vi "Chamber controller June 30 2016 TEMP.vi"() -> ()   [LabVIEW 2014]
uses:
  <vilib>/Instr/_visa.llb/VISA Configure Serial Port (Instr).vi
  Environmental Chamber LabVIEW and Instruments/Drivers and Software/Keithley 2100 Series/Public/Configure/Configure 2 Wire Resistance.vi
  <vilib>/Utility/file.llb/Write To Spreadsheet File (string).vi
  <vilib>/Utility/file.llb/Read From Spreadsheet File (string).vi
  Environmental Chamber LabVIEW and Instruments/Drivers and Software/keithley_6430/Keithley 6430/Public/Data/Read (Single Point).vi
  Environmental Chamber LabVIEW and Instruments/Drivers and Software/LabVIEW 8.2 Drivers/keithley_24xx/Keithley 24XX/Public/Data/Read (Single Point).vi
  Environmental Chamber LabVIEW and Instruments/Drivers and Software/keithley_24xx/Keithley 24XX/Keithley 24XX.lvlib
  Environmental Chamber LabVIEW and Instruments/Drivers and Software/keithley_6430/Keithley 6430/Keithley 6430.lvlib
  Environmental Chamber LabVIEW and Instruments/Drivers and Software/Keithley 2100 Series/Keithley 2100 Series.lvlib
panel:
  out "Current setpoint (C)":dbl
  in  "J-KEM temp control cluster":T1 {"Set temp (C)" min=0.0 max=130.0}
  out "saving data?":bool
  out "ArduinoQCM\ncluster":T2 caption="Arduino QCM" {"Freq 5" format="%#_10g"; "Freq 4" format="%#_10g"; "Freq 3" format="%#_10g"; "Freq 2" format="%#_10g"; "Freq 1" format="%#_10g"}
  in  "Data logging settings":T3={"Save during sequence only"=TRUE, "Save now"=FALSE, "sec between data points"=0.0, "Current data file path"=path "", "Save sample names"={"QCM1"="aQCM2", "QCM2"="aQCM2", "QCM3"="aQCM3", "QCM4"="aQCM4", "QCM5"="aQCM5", "QCM6"="aQCM6", "SRS"="sample_SRS", "K-2420"="Keithley2420", "K-6430"="Keithley6430", "K-2100"="Keithley2100"}, "Experiment Notes"=""} {"sec between data points" min=0.0 max=30.0 format="%#_13g"}
  in  "Sequence cluster":T4={"Save sequence"=FALSE, "Clear sequence"=FALSE, "Import sequence file"=FALSE, "Tare elapsed time"=TRUE, "Run Sequence"=FALSE, "Stop program when sequence ends"=TRUE, "User-defined\nsequence"=[], "Sequence end time"="", "Sequence\npreview"=[]} caption="Sequence settings"
  in  "Pressure parameters cluster":T5={"valve % open"=100.0, "Desired pressure"=0.0, "Vapor sccm"=0.0, "Gas sccm"=0.0, "Valve mode"=enum."% Open", "Pressure Mode"=enum."Abs. pressure", "analyte partial pressure"=23.8, "Turbo pump\nauto on"=TRUE, "Valve position (%)"=0.0, "read pressure"=0.0, "read vapor flow"=0.0, "read gas flow"=0.0, "pressure chart"={"pressure"=0.0}} caption="Pressure settings" {"read gas flow" format="%#_3g"; "read vapor flow" format="%#_3g"; "read pressure" format="%#_7f"; "Valve position (%)" format="%#_3g"; "analyte partial pressure" min=0.0 max=100.0 step=5.0; "Gas sccm" min=0 max=200 step=5; "Vapor sccm" min=0 max=200 step=5; "Desired pressure" min=0.0 max=760.0 step=5.0; "valve % open" min=0.0 max=100.0 step=5.0 format="%#_2f"}
  out "Elapsed time (min)":dbl
  out "State date/time":string caption="Start time"
  out "K-2100 (Ohm)":cluster{"Measurement":dbl}(graph) caption="K-2100 Ohm"
  out "K-6430":cluster{"Measurement":dbl}(graph)
  out "K-2420":cluster{"Resistance":sgl}(graph)
  in  "Gate time (sec)":enum16{"0.1", "1.0 ", "10"}(ring)=enum."1.0 "
  out "MHz":dbl format="%.9f"
  out "QCM plot":T6(graph)
  in  "Stop":bool
  in  "Clear all charts":bool
  out "O2 sensor output":dbl[](array[numeric]) caption="atm\nTorr"
  in  "rapidox O2 Sensor":bool
  in  "setnag O2 Pump":bool
  in  "Baud Rate 2":i32(ring)=2 items=["2400", "4800", "9600", "19200", "38400", "57600", "115200"]
  in  "Com Port":i32(ring) items=["Com 1", "Com 2", "Com 3", "Com 4", "Com 5", "Com 6", "COM 7", "COM 8", "COM 9", "COM 10", "COM 11", "COM 12", "com 13", "COM 14"]
  in  "Com Port 2":i32(ring) items=["Com 1", "Com 2", "Com 3", "Com 4", "Com 5", "Com 6", "COM 7", "COM 8", "COM 9", "COM 10", "COM 11", "COM 12", "com 13", "COM 14"]
  out "Waveform Chart":cluster{dbl}(graph)
  out "O2 Concentration (PPM)":dbl
  out "Waveform Chart 6":cluster{dbl}(graph)
  # "Currently Unused"
  # "100%"
  # "SRS"
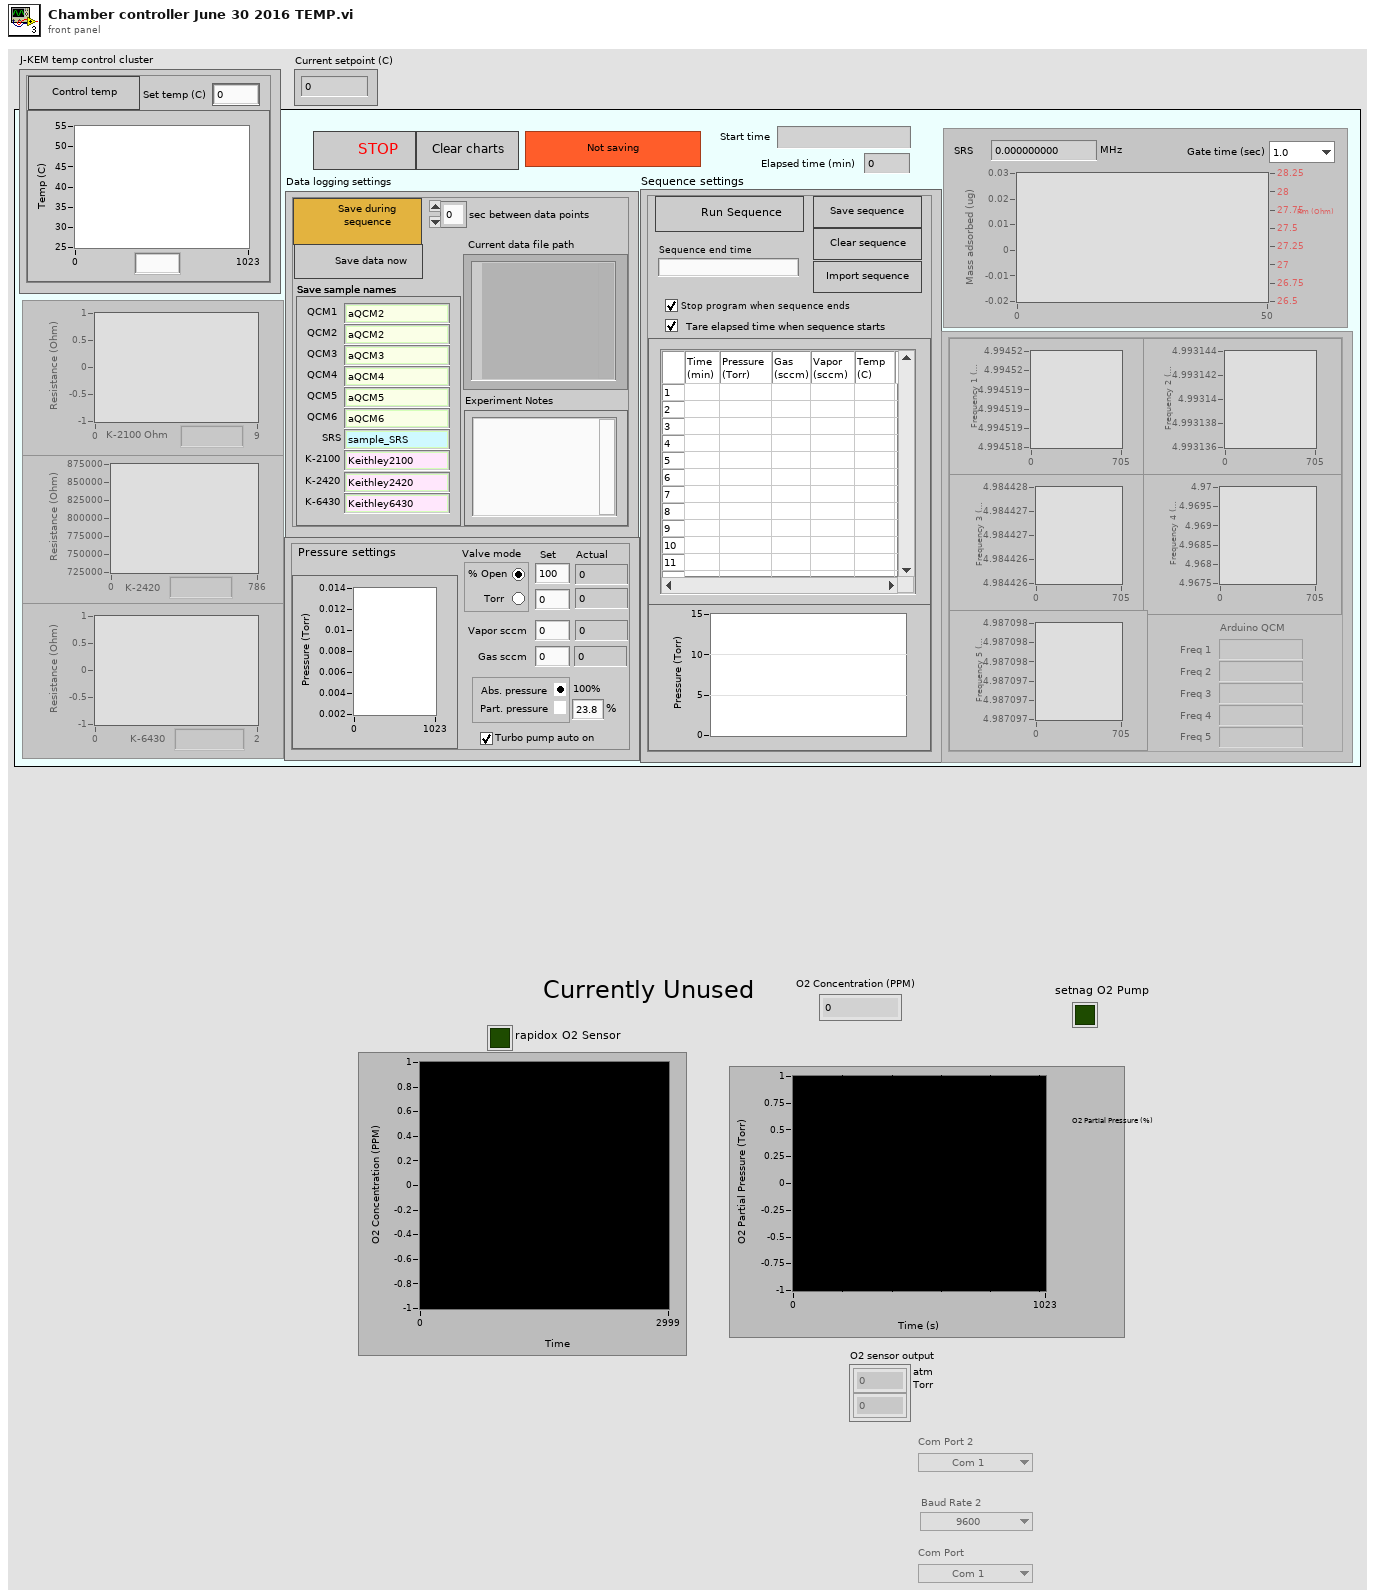
[diagram p1: front panel]
types:
  T1 = cluster{"Set temp (C)":dbl, "Control temp":bool, "J-KEM temp chart":dbl}
  T2 = cluster{"arduino qcm 1":dbl, "Freq 1":dbl, "arduino qcm 2":dbl, "Freq 2":dbl, "arduino qcm 3":dbl, "Freq 3":dbl, "arduino qcm 4":dbl, "Freq 4":dbl, "arduino qcm 5":dbl, "Freq 5":dbl}
  T3 = cluster{"Save during sequence only":bool, "Save now":bool, "sec between data points":dbl, "Current data file path":path, "Save sample names":cluster{"QCM1":string, "QCM2":string, "QCM3":string, "QCM4":string, "QCM5":string, "QCM6":string, "SRS":string, "K-2420":string, "K-6430":string, "K-2100":string}, "Experiment Notes":string}
  T4 = cluster{"Save sequence":bool, "Clear sequence":bool, "Import sequence file":bool, "Tare elapsed time":bool, "Run Sequence":bool, "Stop program when sequence ends":bool, "User-defined\nsequence":string[][], "Sequence end time":string, "Sequence\npreview":cluster{dbl[], dbl[]}[]}
  T5 = cluster{"valve % open":dbl, "Desired pressure":dbl, "Vapor sccm":sgl, "Gas sccm":sgl, "Valve mode":enum32{"% Open", "Torr "}, "Pressure Mode":enum32{"Abs. pressure", " Part. pressure"}, "analyte partial pressure":dbl, "Turbo pump\nauto on":bool, "Valve position (%)":dbl, "read pressure":dbl, "read vapor flow":dbl, "read gas flow":dbl, "pressure chart":cluster{"pressure":dbl}}
  T6 = cluster{"Numeric Control":dbl, "Resistance out":dbl}
  T7 = cluster{"Keithley 6430":bool, "J-KEM":bool, "Keithley 2420":bool, "Keithley 2100":bool, "SRS QCM":bool, "Pressure control":bool, "Arduino":bool}
  T8 = enum8{"Enabled", "Disabled", "Disabled and Grayed Out"}
  T9 = cluster{"Arduino 1":refnum<visa-resource-name>, "Arduino 2":refnum<visa-resource-name>, "Arduino 3":refnum<visa-resource-name>, "Arduino 4":refnum<visa-resource-name>, "Arduino 5":refnum<visa-resource-name>}
  T10 = enum16{"open", "open or create", "create or replace", "create", "open (read only)"}
  T11 = enum16{"no parity", "odd parity", "even parity", "mark parity", "space parity"}
  T12 = cluster{"f":dbl, "f":dbl, "f":dbl, "f":dbl, "f":dbl}
  T13 = cluster{"String":string, "String":string, "String":string}
  T14 = cluster{"task out":refnum<k21>, "error out":errorcluster, "task out":refnum<k21>, "error out":errorcluster, "task out":refnum<k21>, "error out":errorcluster, "VISA resource name":refnum<visa-resource-name>, "error out":errorcluster}
  T15 = cluster{"task out":refnum<k21>, "error out":errorcluster, "task out":refnum<k21>, "error out":errorcluster, "task out":refnum<k21>, "error out":errorcluster, "VISA resource name out":refnum<visa-resource-name>, "error out":errorcluster}
  T16 = cluster{bool, "VISA resource name":refnum<visa-resource-name>, "error out":errorcluster}
  T17 = cluster{bool, "VISA resource name out":refnum<visa-resource-name>, "error out":errorcluster}
  T18 = cluster{"VISA resource name out":refnum<visa-resource-name>, "error out":errorcluster, "VISA resource name out":refnum<visa-resource-name>, "error out":errorcluster, "VISA resource name out":refnum<visa-resource-name>, "error out":errorcluster, "VISA resource name out":refnum<visa-resource-name>, "error out":errorcluster, "VISA resource name out":refnum<visa-resource-name>, "error out":errorcluster}
  T19 = cluster{bool, cluster{"task out":refnum<k21>, "error out":errorcluster, "task out":refnum<k21>, "error out":errorcluster, "task out":refnum<k21>, "error out":errorcluster, "VISA resource name out":refnum<visa-resource-name>, "error out":errorcluster}}
  T20 = cluster{bool, "VISA out":refnum<visa-resource-name>, "error out":errorcluster}
  T21 = cluster{"Boolean":bool, "VISA out":refnum<visa-resource-name>, "error out":errorcluster}
  T22 = cluster{"Numeric Control":dbl, "Cluster":cluster{"Numeric Control":dbl}, "String":string, "error out":errorcluster}
  T23 = cluster{bool, "Com Port":i32, "Numeric Control out":dbl}
  T24 = cluster{"VISA Refnum out":refnum<visa-resource-name>, "error out":errorcluster, "VISA Refnum out":refnum<visa-resource-name>, "error out":errorcluster, "VISA Refnum out":refnum<visa-resource-name>, "error out":errorcluster, "VISA Refnum out":refnum<visa-resource-name>, "error out":errorcluster, "VISA Refnum out":refnum<visa-resource-name>, "error out":errorcluster}
  T25 = cluster{"f":string, "f":string, "f":string, "f":string, "f":string}
  T26 = cluster{"valve % open":dbl, "Desired pressure":dbl, "Vapor sccm":sgl, "Gas sccm":sgl, "Valve mode":enum32{"% Open", "Torr "}, "Pressure Mode":enum32{"Abs. pressure", " Part. pressure"}, "analyte partial pressure":dbl, "Turbo pump\nauto on":bool}
  T27 = cluster{"User-defined\nsequence":string[][], "Present (s)":dbl, "current  step # in":i32, "sequence end time in":timestamp}
  T28 = cluster{"current  step # in":i32, "sequence end time in":timestamp, "Boolean":bool}
  T29 = cluster{"press/RH/gas/vapor":cluster{"pressure":string, "RH":string, "gas flow":string, "vapor flow":string}, "Cluster":cluster{"Valve position (%)":dbl, "read pressure":dbl, "read vapor flow":dbl, "read gas flow":dbl}}
  T30 = cluster{"Boolean":bool, "DAQ IDs in":cluster{"task out":refnum<k21>, "error out":errorcluster, "task out":refnum<k21>, "error out":errorcluster, "task out":refnum<k21>, "error out":errorcluster, "VISA Refnum out":refnum<visa-resource-name>, "error out":errorcluster}}
  T31 = cluster{"Boolean":bool, "VISA resource name out":refnum<visa-resource-name>, "error out":errorcluster}
  T32 = cluster{"current temp string":string, string, string, string}
  T33 = cluster{"f":dbl, "f":dbl, "f":dbl, "f":dbl, "f":dbl}[]
  T34 = cluster{"pressure":string, "RH":string, "gas flow":string, "vapor flow":string}
  T35 = cluster{"Valve position (%)":dbl, "read pressure":dbl, "read vapor flow":dbl, "read gas flow":dbl}
  T36 = cluster{"f":dbl, "f":dbl, "f":dbl, "f":dbl, "f":dbl, "f":dbl, "f":dbl, "f":dbl, "f":dbl, "f":dbl}
  T37 = cluster{"QCM1":string, "QCM2":string, "QCM3":string, "QCM4":string, "QCM5":string, "QCM6":string, "SRS":string, "K-2420":string, "K-6430":string, "K-2100":string}
  T38 = cluster{"task out":refnum<k21>, "error out":errorcluster, "task out":refnum<k21>, "error out":errorcluster, "task out":refnum<k21>, "error out":errorcluster, "VISA Refnum out":refnum<visa-resource-name>, "error out":errorcluster}
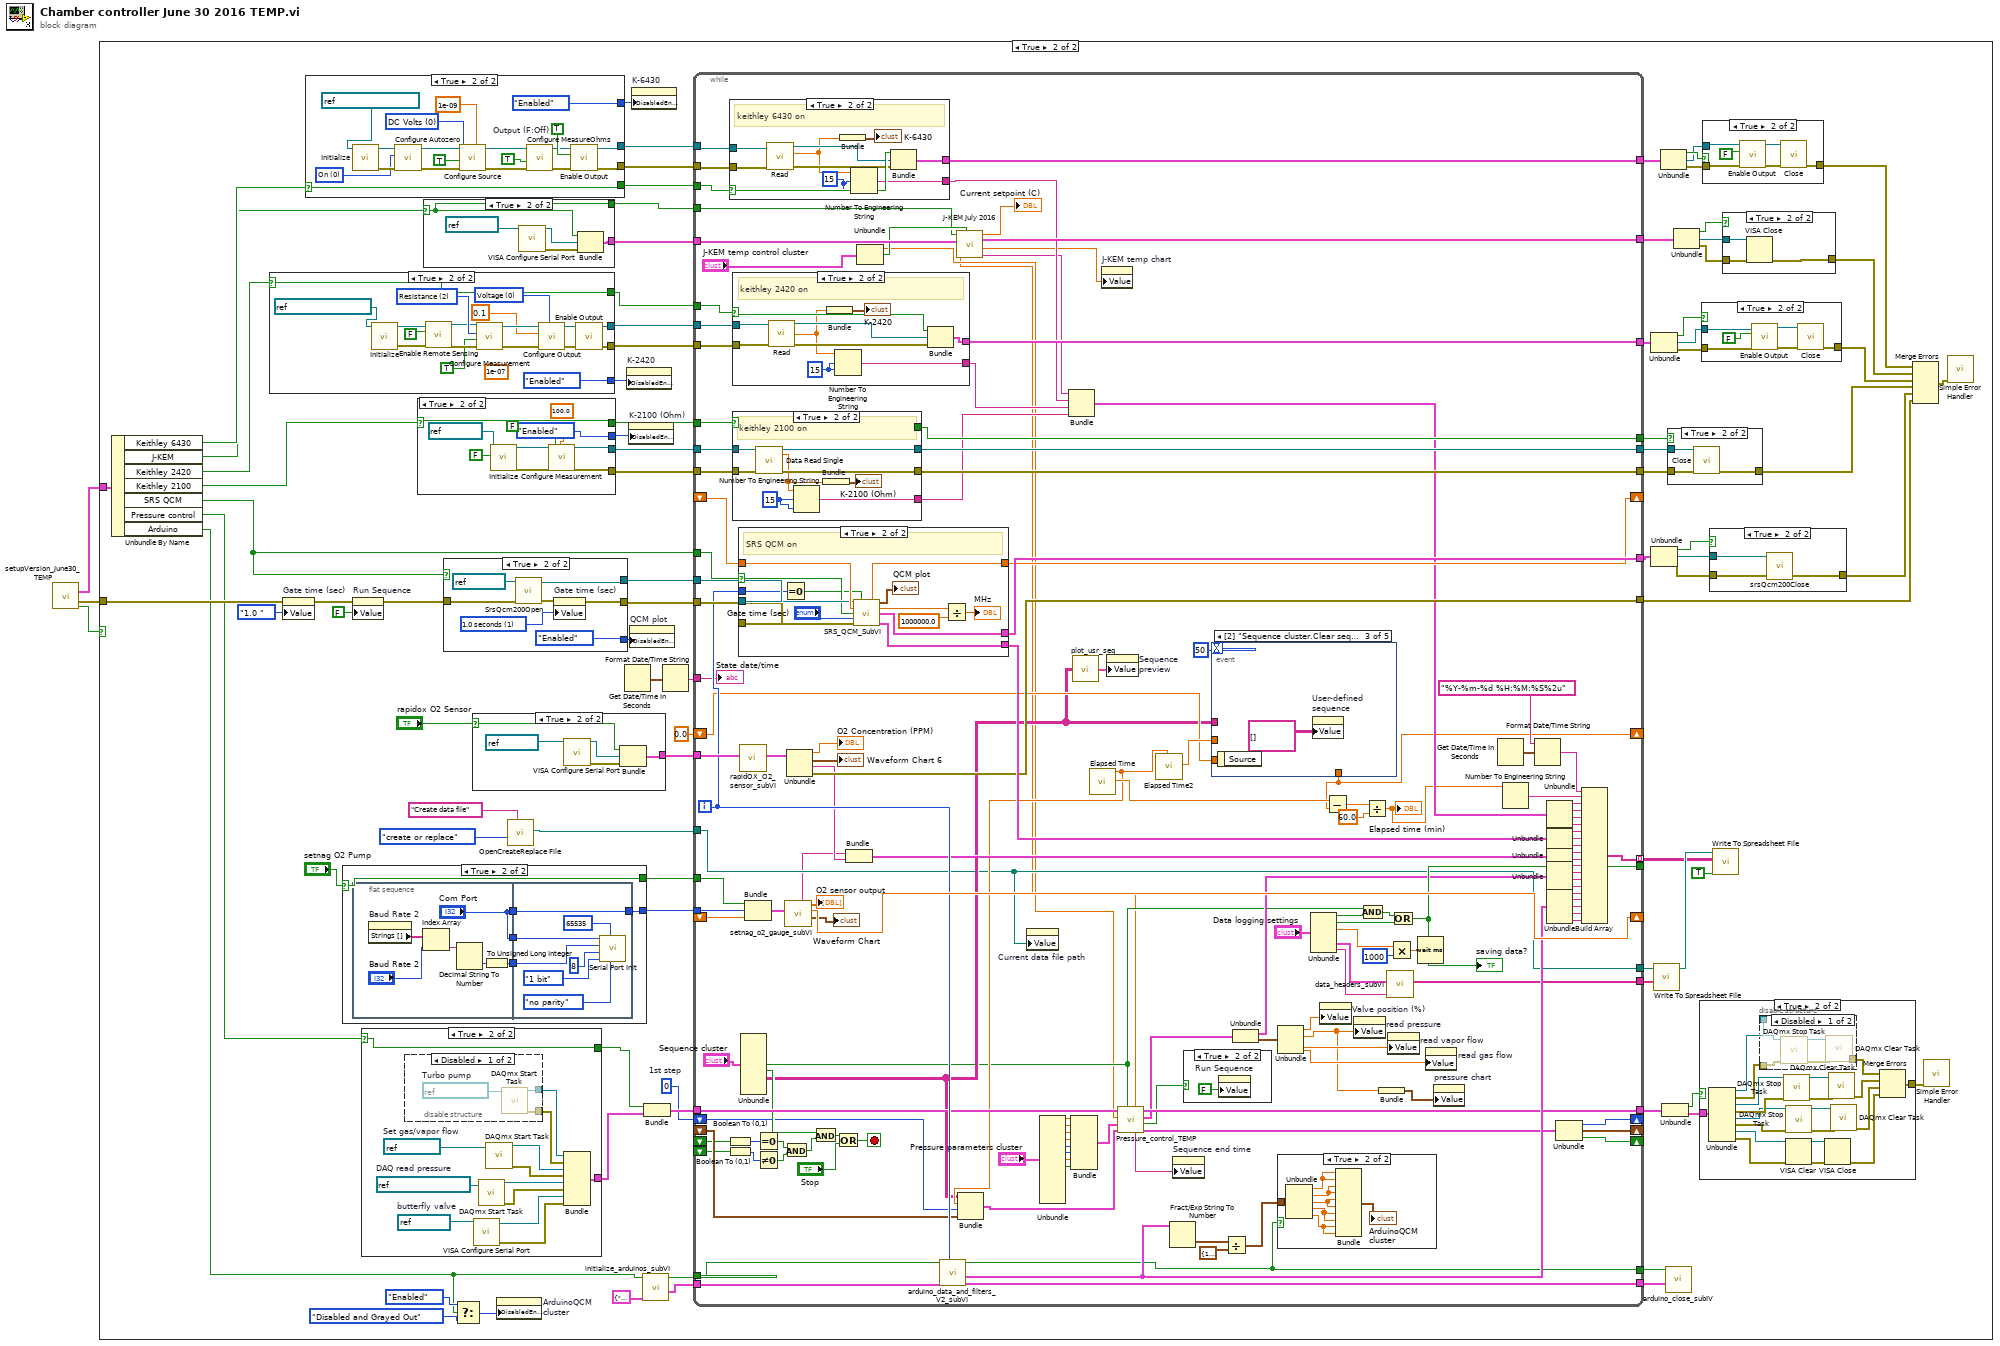
[diagram p0: block diagram]
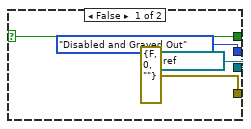
[diagram p4: hidden frame]
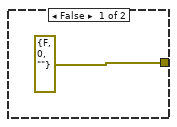
[diagram p5: hidden frame]
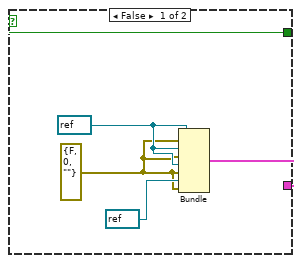
[diagram p7: hidden frame]
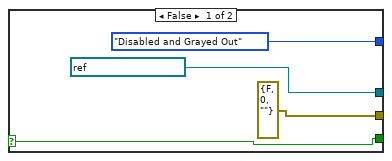
[diagram p10: hidden frame]
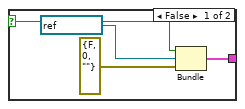
[diagram p11: hidden frame]
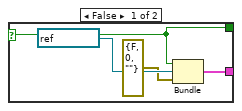
[diagram p13: hidden frame]
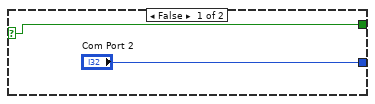
[diagram p14: hidden frame]
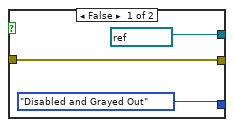
[diagram p16: hidden frame]
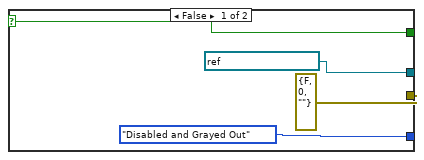
[diagram p18: hidden frame]
diagram:
  n1 = call "setupVersion_June30_TEMP.vi"() -> ("Instruments on/off"=w1:T7, "error IO"=w2:errorcluster, "OK"=w3:bool)  [unwired: 13 in]
  n2 = case shown="True" w3 {
    tunnel: w2 -> [_ w12]
    tunnel: w1 -> [_ w11]
    frame False {
    }
    frame True {
      w24 = 0  # 1st step
      n3 = Unbundle By Name(w11) -> ("Keithley 6430"=w10:bool, "J-KEM"=w9:bool, "Keithley 2420"=w8:bool, "Keithley 2100"=w7:bool, "SRS QCM"=w6:bool, "Pressure control"=w5:bool, "Arduino"=w4:bool)
      n4 = case shown="True" w8 {
        selector: w8 -> [w250 w254]
        tunnel: [refnum<visa-resource-name> "GPIB1::24::INSTR" ("VISA resource name") w263] -> w89
        tunnel: [errorcluster {"status"=FALSE, "code"=0, "source"=""} ("error out") w258] -> w88
        tunnel: [T8."Disabled and Grayed Out" ("Disabled") T8."Enabled" ("Disabled")] -> w52
        tunnel: [w250 w254] -> w45
        frame False {
        }
        frame True {
          (unwired) 1e-07 ("Manual Range (1.0)")
          w265 = u16 0 items=["Voltage", "Current"] ("Source Mode  (0: Voltage)")
          w270 = u16 2 items=["Volts", "Current", "Resistance"] ("Function (0: Volts)")
          n5 = call "Initialize.vi"("VISA resource name"=refnum<visa-resource-name> "GPIB1::24::INSTR") -> ("error out"=w259:errorcluster, "VISA resource name out"=w262:refnum<visa-resource-name>)  [unwired: 9 in]
          n6 = call "Enable Remote Sensing.vi"("error in (no error)"=w259, "Enable Remote Sensing (T: Enable)"=FALSE ("4-wire?"), "VISA resource name"=w262) -> ("error out"=w260:errorcluster, "VISA resource name out"=w261:refnum<visa-resource-name>)  [unwired: 7 in]
          n7 = call "Configure Measurement.vi"("error in (no error)"=w260, "Enable Auto Range (T:Enable)"=TRUE, "Function (0: Volts)"=w270, "VISA resource name"=w261) -> ("error out"=w269:errorcluster, "VISA resource name out"=w268:refnum<visa-resource-name>)  [unwired: 6 in]
          n8 = call "Configure Output.vi"("Source Mode  (0: Voltage)"=w265, "error in (no error)"=w269, "Output Level (0)"=0.1 ("Applied Voltage (V)"), "VISA resource name"=w268) -> ("error out"=w267:errorcluster, "VISA resource name out"=w266:refnum<visa-resource-name>)  [unwired: 6 in]
          n9 = call "Enable Output.vi"("error in (no error)"=w267, "VISA resource name"=w266) -> ("error out"=w258:errorcluster, "VISA resource name out"=w263:refnum<visa-resource-name>)  [unwired: 8 in]
        }
      }
      n10 = property on="Gate time (sec)" class="Enum (strict)"(error in=w12, "Value"=enum16{"0.1", "1.0 ", "10"}."1.0 " ("Gate time (sec)")) -> (error out=w13:errorcluster)  [unwired: 1 in, 1 out]
      n11 = case shown="True" w10 {
        selector: w10 -> [w164 w168]
        tunnel: [refnum<visa-resource-name> "GPIB0::29::INSTR" ("VISA resource name") w181] -> w58
        tunnel: [errorcluster {"status"=FALSE, "code"=0, "source"=""} ("error out") w182] -> w57
        tunnel: [T8."Disabled and Grayed Out" ("Disabled") T8."Enabled" ("Disabled")] -> w51
        tunnel: [w164 w168] -> w44
        frame False {
        }
        frame True {
          w170 = u16 0 items=["DC Volts", "DC Current"] ("Source Function (0: DC Volts)")
          w177 = u16 0 items=["On", "Off", "Once"] ("Autozero  (0: On)")
          w185 = TRUE  # Output (F:Off)
          n12 = call "Initialize.vi"("VISA resource name"=refnum<visa-resource-name> "GPIB0::30::INSTR") -> ("error out"=w178:errorcluster, "VISA resource name out"=w179:refnum<visa-resource-name>)  [unwired: 4 in, 5 out]
          n13 = call "Configure Autozero.vi"("error in (no error)"=w178, "Autozero  (0: On)"=w177, "VISA resource name"=w179) -> ("error out"=w173:errorcluster, "VISA resource name out"=w175:refnum<visa-resource-name>)  [unwired: 7 in]
          n14 = call "Configure Source.vi"("I-Source Level [A]"=1e-09, "error in (no error)"=w173, "Auto Range (T:Enable)"=TRUE, "Source Function (0: DC Volts)"=w170, "VISA resource name"=w175) -> ("error out"=w172:errorcluster, "VISA resource name out"=w174:refnum<visa-resource-name>)  [unwired: 5 in]
          n15 = call "Configure MeasureOhms.vi"("error in (no error)"=w172, "Auto Range (T:Enable)"=TRUE, "VISA resource name"=w174) -> ("error out"=w186:errorcluster, "VISA resource name out"=w184:refnum<visa-resource-name>)  [unwired: 3 in, 4 out]
          n16 = call "Enable Output.vi"("error in (no error)"=w186, "Enable Output (F:Off)"=w185, "VISA resource name"=w184) -> ("error out"=w182:errorcluster, "VISA resource name out"=w181:refnum<visa-resource-name>)  [unwired: 7 out]
        }
      }
      n17 = case shown="True" "setnag O2 Pump" {
        selector: "setnag O2 Pump" -> [w209 w211]
        tunnel: ["Com Port 2" w212] -> w85
        tunnel: [w209 w211] -> w33
        frame False {
        }
        frame True {
          n18 = flat-sequence {
            tunnel: ["Com Port"] -> w215
            tunnel: [w217] -> w214
            tunnel: ["Com Port"] -> w213
            tunnel: w215 -> [w223]
            tunnel: w214 -> [w222]
            tunnel: w213 -> [w224]
            tunnel: [w224] -> w212
            frame #0 {
              n19 = property on="Baud Rate 2" class="Ring (strict)"() -> ("Strings []"=w219:string[])  [unwired: 2 in, 2 out]
              n20 = Index Array(array=w219, index="Baud Rate 2") -> (element=w220:string)
              n21 = Decimal String To Number(string=w220) -> (number=w218:i32)  [unwired: 2 in, 1 out]
              n22 = To Unsigned Long Integer(number=w218) -> (unsigned 32bit integer=w217:u32)
            }
            frame #1 {
              n23 = call <vilib>:"Serial Port Init.vi"("parity"=T11."no parity", "buffer size"=u16 65535, "stop bits"=enum16{"1 bit", "1.5 bits", "2 bits"}."1 bit", "data bits"=u16 8, "baud rate"=w222, "port number"=w223) -> ()  [unwired: 1 in, 1 out]
            }
          }
        }
      }
      n24 = property on="Run Sequence" class="Bool (strict)"(error in=w13, "Value"=FALSE) -> (error out=w19:errorcluster)  [unwired: 1 in, 1 out]
      n25 = case shown="True" w5 {
        selector: w5 -> [w136 w141]
        tunnel: [w137 w143] -> w26
        tunnel: [w136 w141] -> w27
        frame False {
          w139 = refnum<k21> refnum ("task out")
          w138 = errorcluster {"status"=FALSE, "code"=0, "source"=""} ("error out")
          n26 = Bundle("task out"=w139, "error out"=w138, "task out"=w139, "error out"=w138, "task out"=w139, "error out"=w138, "VISA resource name"=refnum<visa-resource-name> refnum, "error out"=w138) -> (w137:T14)  [unwired: 1 in]
        }
        frame True {
          w151 = refnum<visa-resource-name> "COM5"  # butterfly valve
          w152 = refnum<k21> "Setflow"  # Set gas/vapor flow
          w153 = refnum<k21> "AllDaqReadings"  # DAQ read pressure
          n27 = disable-structure shown="Disabled" {
            disable-tunnel: [w155 _] -> w150
            disable-tunnel: [w154 _] -> w149
            frame Disabled {
              w156 = refnum<k21> "TurboON"  # Turbo pump
              n28 = call <vilib>:"DAQmx Start Task.vi"("task/channels in"=w156) -> ("task out"=w155:refnum<k21>, "error out"=w154:errorcluster)  [unwired: 13 in]
            }
            frame Enabled {
            }
          }
          n29 = call-poly "VISA Configure Serial Port"("VISA resource name"=w151) -> ("VISA resource name out"=w144:refnum<visa-resource-name>, "error out"=w142:errorcluster)  [unwired: 13 in]
          n30 = call <vilib>:"DAQmx Start Task.vi"("task/channels in"=w153) -> ("task out"=w146:refnum<k21>, "error out"=w145:errorcluster)  [unwired: 13 in]
          n31 = call <vilib>:"DAQmx Start Task.vi"("task/channels in"=w152) -> ("task out"=w148:refnum<k21>, "error out"=w147:errorcluster)  [unwired: 13 in]
          n32 = Bundle("task out"=w150, "error out"=w149, "task out"=w148, "error out"=w147, "task out"=w146, "error out"=w145, "VISA resource name out"=w144, "error out"=w142) -> (w143:T15)  [unwired: 1 in]
        }
      }
      n33 = case shown="True" w7 {
        selector: w7 -> [w97 w103]
        tunnel: [refnum<visa-resource-name> "K-2100" ("VISA resource name out") w106] -> w42
        tunnel: [errorcluster {"status"=FALSE, "code"=0, "source"=""} ("error out") w105] -> w41
        tunnel: [w97 w103] -> w40
        tunnel: [T8."Disabled and Grayed Out" ("Disabled") T8."Enabled" ("Disabled")] -> w35
        frame False {
        }
        frame True {
          n34 = call "Initialize.vi"("VISA resource name"=refnum<visa-resource-name> "K-2100", "Reset? (T: Reset)"=FALSE) -> ("VISA resource name out"=w107:refnum<visa-resource-name>, "error out"=w104:errorcluster)  [unwired: 16 in]
          n35 = call-poly "Configure Measurement.vi"("VISA resource name"=w107, "error in (no error)"=w104, "Auto Range? (T: Auto)"=FALSE, "Custom Range (100 Ohm)"=100.0 ("Temp (C) 2")) -> ("VISA resource name out"=w106:refnum<visa-resource-name>, "error out"=w105:errorcluster)  [unwired: 14 in]
        }
      }
      n36 = case shown="True" w9 {
        selector: w9 -> [w200 w205]
        tunnel: [w201 w206] -> w74
        tunnel: [w200 w205] -> w68
        frame False {
          n37 = Bundle(w200, "VISA resource name"=refnum<visa-resource-name> "COM3", "error out"=errorcluster {"status"=FALSE, "code"=0, "source"=""}) -> (w201:T16)  [unwired: 1 in]
        }
        frame True {
          n38 = call-poly "VISA Configure Serial Port"("VISA resource name"=refnum<visa-resource-name> "COM3") -> ("VISA resource name out"=w207:refnum<visa-resource-name>, "error out"=w204:errorcluster)  [unwired: 13 in]
          n39 = Bundle(w205, "VISA resource name out"=w207, "error out"=w204) -> (w206:T17)  [unwired: 1 in]
        }
      }
      n40 = case shown="True" w6 {
        tunnel: [refnum<visa-resource-name> "COM6" ("VISA in") w239] -> w87
        tunnel: [w234 w236] -> w86
        tunnel: w19 -> [w234 w241]
        tunnel: [T8."Disabled and Grayed Out" ("Disabled") T8."Enabled" ("Disabled")] -> w53
        frame False {
        }
        frame True {
          w238 = u16 1 items=["0.1 seconds", "1.0 seconds", "10.0 seconds"] ("Gate time")
          n41 = call "SrsQcm200Open.vi"("error in"=w241, "VISA in"=refnum<visa-resource-name> "COM6") -> ("error out"=w237:errorcluster, "VISA out"=w239:refnum<visa-resource-name>)  [unwired: 3 in]
          n42 = property on="Gate time (sec)" class="Enum (strict)"(error in=w237, "Value"=w238) -> (error out=w236:errorcluster)  [unwired: 1 in, 1 out]
        }
      }
      n43 = Select(t=T8."Enabled" ("Disabled"), s=w4, f=T8."Disabled and Grayed Out" ("Disabled")) -> (s? t:f=w18:T8)
      n44 = case shown="True" "rapidox O2 Sensor" {
        selector: "rapidox O2 Sensor" -> [w187 w192]
        tunnel: [w188 w193] -> w64
        frame False {
          n45 = Bundle(w187, "VISA resource name"=refnum<visa-resource-name> "COM7", "error out"=errorcluster {"status"=FALSE, "code"=0, "source"=""}) -> (w188:T16)  [unwired: 1 in]
        }
        frame True {
          n46 = call-poly "VISA Configure Serial Port"("VISA resource name"=refnum<visa-resource-name> "COM7") -> ("VISA resource name out"=w194:refnum<visa-resource-name>, "error out"=w191:errorcluster)  [unwired: 13 in]
          n47 = Bundle(w192, "VISA resource name out"=w194, "error out"=w191) -> (w193:T17)  [unwired: 1 in]
        }
      }
      n48 = property on="ArduinoQCM\ncluster" class="Clust (strict)"("DisabledEnum"=w18) -> ()  [unwired: 2 in, 2 out]
      n49 = call "OpenCreateReplace File.vi"("prompt"="Create data file", "function (open:0)"=T10."create or replace") -> ("new file path"=w43:path)  [unwired: 6 in, 3 out]
      n50 = Get Date/Time In Seconds() -> (seconds since 1Jan1904=w91:timestamp)
      n51 = property on="K-2420" class="WFChart (strict)"("DisabledEnum"=w52) -> ()  [unwired: 2 in, 2 out]
      n52 = property on="K-2100 (Ohm)" class="WFChart (strict)"("DisabledEnum"=w35) -> ()  [unwired: 2 in, 2 out]
      n53 = property on="QCM plot" class="WFChart (strict)"("DisabledEnum"=w53) -> ()  [unwired: 2 in, 2 out]
      n54 = property on="K-6430" class="WFChart (strict)"("DisabledEnum"=w51) -> ()  [unwired: 2 in, 2 out]
      n55 = call "initialize_arduinos_subVI.vi"("arduino 1-6 addresses"=T9 {"Arduino 1"="COM21", "Arduino 2"="COM22", "Arduino 3"="COM23", "Arduino 4"="COM24", "Arduino 5"="COM26"}, "arduinos on?"=w4) -> ("arduino addresses/errors"=w28:T18, "arduinos on/off"=w49:bool)  [unwired: 8 in]
      n56 = Bundle(w27, w26) -> (w25:T19)  [unwired: 1 in]
      n57 = Format Date/Time String(seconds (now)=w91) -> (date/time string=w32:string)  [unwired: 2 in]
      n58 = while {
        shift-right: [w418] -> _
        shift-left: _ -> [w340]
        tunnel: [w403] -> w50 mode=indexing if=w366
        tunnel: w45 -> [w408]
        tunnel: w89 -> [w417]
        tunnel: w88 -> [w416]
        tunnel: w87 -> [w415]
        tunnel: w86 -> [w414]
        tunnel: w6 -> [w413]
        tunnel: w33 -> [w342]
        tunnel: w85 -> [w343]
        tunnel: [w412] -> w82
        tunnel: [w411] -> w78
        tunnel: w74 -> [w410]
        tunnel: [w409] -> w73
        tunnel: w68 -> [w275]
        tunnel: w64 -> [w354]
        tunnel: [w350] -> w30
        tunnel: [w282] -> w63
        tunnel: w43 -> [w282]
        shift-right: [w401] -> _
        shift-left: _ -> [w402]
        tunnel: w58 -> [w407]
        tunnel: w57 -> [w406]
        tunnel: [w405] -> w56
        tunnel: [w366] -> _
        tunnel: w49 -> [w349]
        tunnel: w28 -> [w394]
        tunnel: [w348] -> w47
        tunnel: [w393] -> w48
        tunnel: [w385] -> w46
        tunnel: w44 -> [w378]
        tunnel: w42 -> [w365]
        tunnel: w41 -> [w364]
        tunnel: w40 -> [w363]
        tunnel: [w362] -> w39
        tunnel: [w361] -> w38
        tunnel: [w360] -> w37
        shift-right: [w334] -> _
        shift-left: 0.0 ("Elapsed Time (s)") -> [w335]
        tunnel: w32 -> [w325]
        tunnel: w25 -> [w307]
        shift-right: [w302] -> _
        shift-left: w24 -> [w295]
        shift-right: [w301] -> _
        shift-left: _ -> [w299]
        shift-right: [w300] -> _
        shift-left: _ -> [w298]
        shift-left: _ -> [w297]
        tunnel: [w293] -> w23
        i -> [w344]
        stop <- w368 stop-if-true
        n59 = Boolean To (0,1)(Boolean=w298) -> (0, 1=w376:i16)
        n60 = Boolean To (0,1)(Boolean=w297) -> (0, 1=w375:i16)
        n61 = case "Keithley 6430" shown="True" w378 {
          selector: w378 -> [w452 w463]
          tunnel: w407 -> [w451 w460]
          tunnel: w406 -> [w450 w459]
          tunnel: ["" w462] -> w347
          tunnel: [w449 w461] -> w405
          frame False {
            # "keithley 6430 off"
            n62 = Bundle(w452, "VISA resource name out"=w451, "error out"=w450) -> (w449:T17)  [unwired: 1 in]
          }
          frame True {
            w454 = i16 15 ("width (-)")
            # "keithley 6430 on"
            n63 = call-poly "Read.vi"("error in (no error)"=w459, "VISA resource name"=w460) -> ("error out"=w458:errorcluster, "Measurement"=w456:dbl, "VISA resource name out"=w457:refnum<visa-resource-name>)  [unwired: 1 in, 6 out]
            n64 = Bundle("Measurement"=w456) -> (→"K-6430":cluster{"Measurement":dbl})  [unwired: 1 in]
            n65 = Number To Engineering String(2:w454, 3:w454, 4:w456) -> (0:w462:string)  [unwired: 1 in]
            n66 = Bundle(w463, "VISA resource name out"=w457, "error out"=w458) -> (w461:T17)  [unwired: 1 in]
          }
        }
        n67 = case shown="True" w363 {
          selector: w363 -> [w428 w433]
          tunnel: [w429 w440] -> w361
          tunnel: [w430 w439] -> w360
          tunnel: w365 -> [w429 w438]
          tunnel: w364 -> [w430 w437]
          tunnel: ["" w435] -> w345
          tunnel: [w428 w433] -> w362
          frame False {
            # "keithley 2100 off"
          }
          frame True {
            w432 = i16 15 ("width (-)")
            # "keithley 2100 on"
            n68 = call "Data Read Single.vi"("VISA resource name"=w438, "error in (no error)"=w437) -> ("VISA resource name out"=w440:refnum<visa-resource-name>, "Measurement"=w436:dbl, "error out"=w439:errorcluster)  [unwired: 15 in]
            n69 = Number To Engineering String ("elapsed time (min)")(2:w432, 3:w432, 4:w436) -> (0:w435:string)  [unwired: 1 in]
            n70 = Bundle("Measurement"=w436) -> (→"K-2100 (Ohm)":cluster{"Measurement":dbl})  [unwired: 1 in]
          }
        }
        n71 = case "Keithley 2420" shown="True" w408 {
          selector: w408 -> [w467 w476]
          tunnel: w417 -> [w466 w471]
          tunnel: w416 -> [w465 w470]
          tunnel: [w464 w474] -> w412
          tunnel: ["" w473] -> w346
          frame False {
            # "keithley 2420 off"
            n72 = Bundle(w467, "VISA resource name out"=w466, "error out"=w465) -> (w464:T17)  [unwired: 1 in]
          }
          frame True {
            w469 = i16 15 ("width (-)")
            # "keithley 2420 on"
            n73 = call-poly "Read.vi"("VISA resource name"=w471, "error in (no error)"=w470) -> ("VISA resource name out"=w477:refnum<visa-resource-name>, "Resistance"=w472:sgl, "error out"=w475:errorcluster)  [unwired: 7 in, 4 out]
            n74 = Bundle("Resistance"=w472) -> (→"K-2420":cluster{"Resistance":sgl})  [unwired: 1 in]
            n75 = Number To Engineering String(2:w469, 3:w469, 4:w472) -> (0:w473:string)  [unwired: 1 in]
            n76 = Bundle(w476, "VISA resource name out"=w477, "error out"=w475) -> (w474:T17)  [unwired: 1 in]
          }
        }
        n77 = case "SRS QCM" shown="True" w413 {
          selector: w413 -> [w481 w492]
          tunnel: w415 -> [w484 w494]
          tunnel: w414 -> [w483 w495]
          tunnel: [w482 w498] -> w411
          tunnel: w402 -> [w479 w497]
          tunnel: [w479 w496] -> w401
          tunnel: [T13 {"String"="", "String"="", "String"=""} ("M,F,MR output cluster") w491] -> w391
          tunnel: w344 -> [_ w485]
          frame False {
            # "SRS QCM off"
            n78 = Bundle(w481, "VISA out"=w484, "error out"=w483) -> (w482:T20)  [unwired: 1 in]
          }
          frame True {
            # "SRS QCM on"
            n79 = Equal To 0?(x=w485) -> (x = 0?=w486:bool)
            n80 = call "SRS_QCM_SubVI.vi"("VISA Refnum in"=w494, "first iteration?"=w486, "Frequency out 3"=w497, "Boolean 2"=w492, "Gate time"="Gate time (sec)", "error in (no error)"=w495) -> ("Frequency out 2"=w496:dbl, "Cluster"=→"QCM plot":T6, "Frequency out"=w487:dbl, "Cluster 2"=w498:T21, "M,F,MR output cluster"=w491:T13)  [unwired: 2 in, 3 out]
            n81 = Divide(x=w487, y=1000000.0) -> (x/y=→"MHz":dbl)
          }
        }
        n82 = call "rapidOX_O2_sensor_subVI.vi"("rapid ox info in"=w354) -> ("rapidox info out"=w353:T22)  [unwired: 10 in]
        n83 = Unbundle("Sequence cluster") -> ("Run Sequence"=w287:bool, "Stop program when sequence ends"=w296:bool, "User-defined\nsequence"=w291:string[][])  [unwired: 6 out]
        n84 = Bundle(w342, "Com Port"=w343, "Numeric Control out"=w340) -> (w341:T23)  [unwired: 1 in]
        n85 = Equal To 0?(x=w376) -> (x = 0?=w373:bool)
        n86 = Not Equal To 0?(x=w375) -> (x != 0?=w374:bool)
        n87 = And(x=w373, y=w374) -> (x .and. y?=w367:bool)
        n88 = call "setnag_o2_gauge_subVI.vi"("setnag info in"=w341) -> ("Cluster"=→"Waveform Chart":cluster{"Numeric Control":dbl}, "Numeric Control out"=w418:dbl, "Array"=→"O2 sensor output":dbl[], "String"=w279:string)  [unwired: 7 in]
        n89 = Unbundle(w353) -> ("Numeric Control"=→"O2 Concentration (PPM)":dbl, "Cluster"=→"Waveform Chart 6":cluster{"Numeric Control":dbl}, "String"=w324:string, "error out"=w350:errorcluster)
        n90 = And(x=w296, y=w367) -> (x .and. y?=w338:bool)
        n91 = Or(x=w338, y="Stop") -> (x .or. y?=w368:bool)
        n92 = Bundle("String"=w279, "String"=w324) -> (w323:cluster{"String":string, "String":string})  [unwired: 1 in]
        n93 = Unbundle("J-KEM temp control cluster") -> ("Set temp (C)"=w273:dbl, "Control temp"=w276:bool)  [unwired: 1 out]
        n94 = call "arduino_data_and_filters_V2_subVI.vi"("loop iteration number"=w344, "arduino 1-6 address and errors"=w394, "arduinos on?"=w349) -> ("arduino 1-6 addresses and errors out"=w393:T24, "arduino 1-6 data out"=w392:T25, "arduinos on? output"=w348:bool)  [unwired: 6 in]
        n95 = property on="Current data file path" class="Path"("Value"=w282) -> ()  [unwired: 2 in, 2 out]
        n96 = Unbundle("Pressure parameters cluster") -> ("valve % open"=w312:dbl, "Desired pressure"=w314:dbl, "Vapor sccm"=w315:sgl, "Gas sccm"=w316:sgl, "Valve mode"=w317:enum32{"% Open", "Torr "}, "Pressure Mode"=w318:enum32{"Abs. pressure", " Part. pressure"}, "analyte partial pressure"=w319:dbl, "Turbo pump\nauto on"=w320:bool)  [unwired: 5 out]
        n97 = Bundle("valve % open"=w312, "Desired pressure"=w314, "Vapor sccm"=w315, "Gas sccm"=w316, "Valve mode"=w317, "Pressure Mode"=w318, "analyte partial pressure"=w319, "Turbo pump\nauto on"=w320) -> (w311:T26)  [unwired: 1 in]
        n98 = call "plot_usr_seq.vi"("User-defined sequence"=w291) -> ("Sequence Preview"=w283:cluster{dbl[], dbl[]}[])
        n99 = call "Elapsed Time"() -> ("Present (s)"=w304:dbl, "Elapsed Time (s)"=w356:dbl)  [unwired: 12 in, 6 out]
        n100 = Bundle("User-defined\nsequence"=w291, "Present (s)"=w304, "current  step # in"=w295, "sequence end time in"=w299) -> (w305:T27)  [unwired: 1 in]
        n101 = property on="Sequence\npreview" class="XYGraph (strict)"("Value"=w283) -> ()  [unwired: 2 in, 2 out]
        n102 = call "Pressure_control_TEMP.vi"("Run Sequence"=w287, "user sequence, present (s) in, current step in, seq time in"=w305, "pressure parameters in"=w311, "set temp"=w273, "pressure control on? / DAQ IDs/errors in"=w307) -> ("current step # out, shift register time out, seq button on?"=w303:T28, "sequence over? USE THIS TO REINITIALIZE RUN SEQUENCE BUTTON SO PROGRAM ENDS"=w292:bool, "save press/RH/gasflow/vaporflow - read valve position/pressure/vaporflow/gasflow"=w290:T29, "pressure control on out, DAQ IDs/errors out"=w293:T30, "sequence end date/time string"=w294:string, "Temp setpoint"=w272:dbl)  [unwired: 1 in]
        n103 = call "J-KEM July 2016.vi"("Control temp?"=w276, "Set temp (C)"=w272, "Address in"=w410, "J-KEM on?"=w275) -> ("current temp string"=w333:string, "Current temp (C)"=w277:dbl, "Address out"=w409:T31, "Current setpoint (C)"=→"Current setpoint (C)":dbl)  [unwired: 4 in]
        n104 = Bundle("current temp string"=w333, w347, w346, w345) -> (w339:T32)  [unwired: 1 in]
        n105 = property on="J-KEM temp chart" class="WFChart (strict)"("Value"=w277) -> ()  [unwired: 2 in, 2 out]
        n106 = call "Elapsed Time2"("Set Start Time (s)"=w304) -> ("Elapsed Time (s)"=w336:dbl)  [unwired: 11 in, 7 out]
        n107 = Fract/Exp String To Number(string=w392) -> (number=w384:T12)  [unwired: 3 in, 1 out]
        n108 = property on="Sequence end time" class="Str"("Value"=w294) -> ()  [unwired: 2 in, 2 out]
        n109 = case shown="True" w292 {
          frame False {
          }
          frame True {
            n110 = property on="Run Sequence" class="Bool (strict)"("Value"=FALSE ("Run Sequence")) -> ()  [unwired: 2 in, 2 out]
          }
        }
        n111 = event shown="[2] \"Sequence cluster.Clear sequence\": Value Change" {
          selector: _ -> [_ _ _ _ _]
          dyn-events: _ -> [_ _ _ _ _]
          timeout: 50 -> [_ _ _ _ _]
          tunnel: w291 -> [_ _ _ w447 _]
          tunnel: w336 -> [_ _ _ _ _]
          tunnel: w335 -> [w441 _ _ _ _]
          tunnel: [w441 _ _ _ _] -> w334
          event Timeout {
            n112 = event-data() -> ()  [unwired: 1 in, 1 out]
          }
          event "Clear all charts": Value Change {
            (unwired) T33 [] ("History Data")
            w444 = cluster{dbl}[] [] ("History Data")
            w445 = cluster{"Resistance":sgl}[] [] ("History Data")
            w443 = dbl[] [] ("History Data")
            n113 = event-data() -> ()  [unwired: 1 in, 1 out]
            n114 = property on="K-6430" class="WFChart (strict)"("History Data"=w445) -> ()  [unwired: 2 in, 2 out]
            n115 = property on="arduino qcm 3" class="WFChart (strict)"("History Data"=w443) -> ()  [unwired: 2 in, 2 out]
            n116 = property on="arduino qcm 1" class="WFChart (strict)"("History Data"=w443) -> ()  [unwired: 2 in, 2 out]
            n117 = property on="Waveform Chart" class="WFChart (strict)"("History Data"=w444) -> ()  [unwired: 2 in, 2 out]
            n118 = property on="QCM plot" class="WFChart (strict)"("History Data"=cluster{dbl, "Resistance out":dbl}[] []) -> ()  [unwired: 2 in, 2 out]
            n119 = property on="K-2100 (Ohm)" class="WFChart (strict)"("History Data"=w445) -> ()  [unwired: 2 in, 2 out]
            n120 = property on="arduino qcm 4" class="WFChart (strict)"("History Data"=w443) -> ()  [unwired: 2 in, 2 out]
            n121 = property on="K-2420" class="WFChart (strict)"("History Data"=w445) -> ()  [unwired: 2 in, 2 out]
            n122 = property on="pressure chart" class="WFChart (strict)"("History Data"=w444) -> ()  [unwired: 2 in, 2 out]
            n123 = property on="arduino qcm 2" class="WFChart (strict)"("History Data"=w443) -> ()  [unwired: 2 in, 2 out]
            n124 = property on="arduino qcm 5" class="WFChart (strict)"("History Data"=w443) -> ()  [unwired: 2 in, 2 out]
          }
          event "Sequence cluster.Clear sequence": Value Change {
            n125 = event-data() -> ()  [unwired: 1 in, 1 out]
            n126 = property on="User-defined\nsequence" class="Tbl (strict)"("Value"=string[][] []) -> ()  [unwired: 2 in, 2 out]
          }
          event "Sequence cluster.Save sequence": Value Change {
            n127 = event-data() -> ()  [unwired: 1 in, 1 out]
            n128 = call-poly <vilib>:"Write To Spreadsheet File.vi"("2D data"=w447) -> ()  [unwired: 7 in, 1 out]
          }
          event "Sequence cluster.Import sequence file": Value Change {
            n129 = event-data() -> ()  [unwired: 1 in, 1 out]
            n130 = call-poly <vilib>:"Read From Spreadsheet File.vi"() -> ("all rows"=w448:string[][])  [unwired: 7 in, 4 out]
            n131 = property on="User-defined\nsequence" class="Tbl (strict)"("Value"=w448) -> ()  [unwired: 2 in, 2 out]
          }
        }
        n132 = Divide(x=w384, y=T12 {"f"=1000000.0, "f"=1000000.0, "f"=1000000.0, "f"=1000000.0, "f"=1000000.0}) -> (x/y=w359:T12)
        n133 = Unbundle(w290) -> ("press/RH/gas/vapor"=w289:T34, "Cluster"=w288:T35)
        n134 = Unbundle(w288) -> ("Valve position (%)"=w286:dbl, "read pressure"=w281:dbl, "read vapor flow"=w285:dbl, "read gas flow"=w284:dbl)
        n135 = case shown="True" w348 {
          tunnel: w359 -> [_ w427]
          frame False {
          }
          frame True {
            n136 = Unbundle(w427) -> ("f"=w426:dbl, "f"=w425:dbl, "f"=w424:dbl, "f"=w423:dbl, "f"=w422:dbl)
            n137 = Bundle("f"=w426, "f"=w426, "f"=w425, "f"=w425, "f"=w424, "f"=w424, "f"=w423, "f"=w423, "f"=w422, "f"=w422) -> (→"ArduinoQCM\ncluster":T36)  [unwired: 1 in]
          }
        }
        n138 = Unbundle("Data logging settings") -> ("Save during sequence only"=w370:bool, "Save now"=w372:bool, "sec between data points"=w358:dbl, "Save sample names"=w309:T37, "Experiment Notes"=w308:string)  [unwired: 1 out]
        n139 = property on="Valve position (%)" class="DigNum (strict)"("Value"=w286) -> ()  [unwired: 2 in, 2 out]
        n140 = Subtract(x=w356, y=w334) -> (x-y=w355:dbl)
        n141 = property on="read pressure" class="DigNum (strict)"("Value"=w281) -> ()  [unwired: 2 in, 2 out]
        n142 = And(x=w287, y=w370) -> (x .and. y?=w369:bool)
        n143 = Divide(x=w355, y=60.0) -> (x/y=w326:dbl)
        "Elapsed time (min)" <- w326
        n144 = Bundle("read pressure"=w281) -> (w280:cluster{"read pressure":dbl})  [unwired: 1 in]
        n145 = call "data_headers_subVI.vi"("Experiment Notes"=w308, "Sample names"=w309) -> ("data headers"=w385:string[])  [unwired: 9 in]
        n146 = property on="read vapor flow" class="DigNum (strict)"("Value"=w285) -> ()  [unwired: 2 in, 2 out]
        n147 = Multiply(x=w358, y=u32 1000 ("x")) -> (x*y=w398:dbl)
        n148 = Or(x=w369, y=w372) -> (x .or. y?=w366:bool)
        "saving data?" <- w366
        n149 = Wait (ms)(milliseconds to wait=w398) -> ()  [unwired: 1 out]
        n150 = property on="read gas flow" class="DigNum (strict)"("Value"=w284) -> ()  [unwired: 2 in, 2 out]
        n151 = property on="pressure chart" class="WFChart (strict)"("Value"=w280) -> ()  [unwired: 2 in, 2 out]
        n152 = Get Date/Time In Seconds() -> (seconds since 1Jan1904=w419:timestamp)
        n153 = Number To Engineering String ("elapsed time (min)")(4:w326) -> (0:w331:string)  [unwired: 3 in]
        n154 = Format Date/Time String(time format string (%c)="%Y-%m-%d %H:%M:%S%2u", seconds (now)=w419) -> (date/time string=w395:string)  [unwired: 1 in]
        n155 = Unbundle(w339) -> ("current temp string"=w330:string, w329:string, w328:string, w327:string)
        n156 = Unbundle(w391) -> ("String"=w332:string, "String"=w397:string, "String"=w396:string)
        n157 = Unbundle(w323) -> ("String"=w322:string, "String"=w321:string)
        n158 = Unbundle(w289) -> ("pressure"=w382:string, "RH"=w381:string, "gas flow"=w380:string, "vapor flow"=w379:string)
        n159 = Unbundle ("arduino 1-6")(w392) -> ("f"=w390:string, "f"=w389:string, "f"=w388:string, "f"=w387:string, "f"=w386:string)
        n160 = Unbundle(w303) -> ("current  step # in"=w302:i32, "sequence end time in"=w301:timestamp, "Boolean"=w300:bool)
        n161 = Build Array(w395, w331, w330, w329, w328, w327, w332, w397, w396, w322, w321, w382, w381, w380, w379, w390, w389, w388, w387, w386) -> (w403:string[])
        "State date/time" <- w325
      }
      n162 = Unbundle(w82) -> (w81:bool, "VISA resource name out"=w80:refnum<visa-resource-name>, "error out"=w79:errorcluster)
      n163 = Unbundle(w78) -> ("Boolean"=w77:bool, "VISA out"=w76:refnum<visa-resource-name>, "error out"=w75:errorcluster)
      n164 = call-poly <vilib>:"Write To Spreadsheet File.vi"("1D data"=w46, "file path (dialog if empty)"=w63) -> ("new file path (Not A Path if cancelled)"=w67:path)  [unwired: 6 in]
      n165 = Unbundle(w56) -> (w61:bool, "VISA resource name out"=w60:refnum<visa-resource-name>, "error out"=w59:errorcluster)
      n166 = Unbundle(w23) -> ("Boolean"=w22:bool, "DAQ IDs in"=w21:T38)
      n167 = call "arduino_close_subIV.vi"("arduino 1-6 addresses and errors out"=w48, "arduinos on?"=w47) -> ()  [unwired: 10 in]
      n168 = case shown="True" w39 {
        tunnel: w38 -> [_ w95]
        tunnel: w37 -> [w92 w94]
        tunnel: [w92 w93] -> w36
        frame False {
        }
        frame True {
          n169 = call "Close.vi"("VISA resource name"=w95, "error in (no error)"=w94) -> ("error out"=w93:errorcluster)  [unwired: 17 in]
        }
      }
      n170 = Unbundle(w73) -> ("Boolean"=w72:bool, "VISA resource name out"=w71:refnum<visa-resource-name>, "error out"=w70:errorcluster)
      n171 = case shown="True" w22 {
        tunnel: w21 -> [_ w124]
        tunnel: [errorcluster {"status"=FALSE, "code"=0, "source"=""} ("error out") w111] -> w31
        frame False {
        }
        frame True {
          n172 = Unbundle(w124) -> ("task out"=w123:refnum<k21>, "error out"=w122:errorcluster, "task out"=w121:refnum<k21>, "error out"=w120:errorcluster, "task out"=w119:refnum<k21>, "error out"=w118:errorcluster, "VISA Refnum out"=w117:refnum<visa-resource-name>, "error out"=w116:errorcluster)
          n173 = disable-structure shown="Disabled" {
            disable-tunnel: [w133 _] -> w115
            disable-tunnel: w123 -> [w132 _]
            disable-tunnel: w122 -> [w131 _]
            frame Disabled {
              n174 = call <vilib>:"DAQmx Stop Task.vi"("task/channels in"=w132, "error in"=w131) -> ("task out"=w134:refnum<k21>, "error out"=w135:errorcluster)  [unwired: 12 in]
              n175 = call <vilib>:"DAQmx Clear Task.vi"("task in"=w134, "error in"=w135) -> ("error out"=w133:errorcluster)  [unwired: 13 in]
            }
            frame Enabled {
            }
          }
          n176 = call <vilib>:"DAQmx Stop Task.vi"("task/channels in"=w121, "error in"=w120) -> ("task out"=w128:refnum<k21>, "error out"=w127:errorcluster)  [unwired: 12 in]
          n177 = call <vilib>:"DAQmx Stop Task.vi"("task/channels in"=w119, "error in"=w118) -> ("task out"=w129:refnum<k21>, "error out"=w130:errorcluster)  [unwired: 12 in]
          n178 = VISA Clear(VISA resource name=w117, error in (no error)=w116) -> (VISA resource name out=w126:refnum<visa-resource-name>, error out=w125:errorcluster)
          n179 = VISA Close(VISA resource name=w126, error in (no error)=w125) -> (error out=w112:errorcluster)
          n180 = call <vilib>:"DAQmx Clear Task.vi"("task in"=w128, "error in"=w127) -> ("error out"=w114:errorcluster)  [unwired: 13 in]
          n181 = call <vilib>:"DAQmx Clear Task.vi"("task in"=w129, "error in"=w130) -> ("error out"=w113:errorcluster)  [unwired: 13 in]
          n182 = Merge Errors(w115, w114, w113, w112) -> (w111:errorcluster)
        }
      }
      n183 = case shown="True" w81 {
        tunnel: w80 -> [_ w246]
        tunnel: w79 -> [w243 w245]
        tunnel: [w243 w244] -> w83
        frame False {
        }
        frame True {
          n184 = call "Enable Output.vi"("error in (no error)"=w245, "Enable Output (T: Enable)"=FALSE, "VISA resource name"=w246) -> ("error out"=w247:errorcluster, "VISA resource name out"=w249:refnum<visa-resource-name>)  [unwired: 7 in]
          n185 = call "Close.vi"("error in (no error)"=w247, "VISA resource name"=w249) -> ("error out"=w244:errorcluster)  [unwired: 9 in]
        }
      }
      n186 = case shown="True" w61 {
        tunnel: w60 -> [_ w159]
        tunnel: w59 -> [w157 w158]
        tunnel: [w157 w160] -> w55
        frame False {
        }
        frame True {
          n187 = call "Enable Output.vi"("error in (no error)"=w158, "Enable Output (F:Off)"=FALSE ("Output (F:Off)"), "VISA resource name"=w159) -> ("error out"=w161:errorcluster, "VISA resource name out"=w162:refnum<visa-resource-name>)  [unwired: 7 out]
          n188 = call "Close.vi"("error in (no error)"=w161, "VISA resource name"=w162) -> ("error out"=w160:errorcluster)  [unwired: 9 out]
        }
      }
      n189 = case shown="True" w77 {
        tunnel: w75 -> [w229 w232]
        tunnel: [w229 w231] -> w84
        tunnel: w76 -> [_ w230]
        frame False {
        }
        frame True {
          n190 = call "srsQcm200Close.vi"("error in"=w232, "Visa in"=w230) -> ("error out"=w231:errorcluster)  [unwired: 3 in]
        }
      }
      n191 = call-poly <vilib>:"Write To Spreadsheet File.vi"("append to file? (new file:F)"=TRUE, "2D data"=w50, "file path (dialog if empty)"=w67) -> ()  [unwired: 5 in, 1 out]
      n192 = case shown="True" w72 {
        tunnel: w71 -> [_ w199]
        tunnel: w70 -> [w196 w198]
        tunnel: [w196 w197] -> w69
        frame False {
        }
        frame True {
          n193 = VISA Close(VISA resource name=w199, error in (no error)=w198) -> (error out=w197:errorcluster)
        }
      }
      n194 = Merge Errors(w55, w69, w83, w36, w84, w30) -> (w90:errorcluster)
      n195 = call <vilib>:"Simple Error Handler.vi"("error in (no error)"=w31) -> ()  [unwired: 4 in, 5 out]
      n196 = call <vilib>:"Simple Error Handler.vi"("error in (no error)"=w90) -> ()  [unwired: 4 in, 5 out]
    }
  }
